vi "Autonomous.vi"   [LabVIEW 2019]
doc: "This VI starts when autonomous period begins, and will automatically be terminated when it ends. You can carry out timed or sensor driven operations directly to I/O or to subsystems without needing to return to the caller."
uses:
  <vilib>/Rock Robotics/WPI/Utilities/WPI_GetSetVariantRefNum.vi
  <vilib>/Rock Robotics/Network Tables/NT Read String.vi
types:
  T1 = typedef "WPI_JoystickDevRef.ctl" = cluster{"Device":T2}
  T2 = typedef "WPI_JoystickDeviceEnum.ctl" = enum16{"USB 0", "USB 1", "USB 2", "USB 3", "USB 4", "USB 5"}
  T3 = typedef "Command Status Info.ctl" = cluster{"Name":string, "Status":T4, "notifier out":T5}
  T4 = typedef "Completion Status.ctl" = enum16{"Successful", "Aborted", "Incomplete"}
  T5 = typedef "Completion Notifier.ctl" = refnum<notifier>
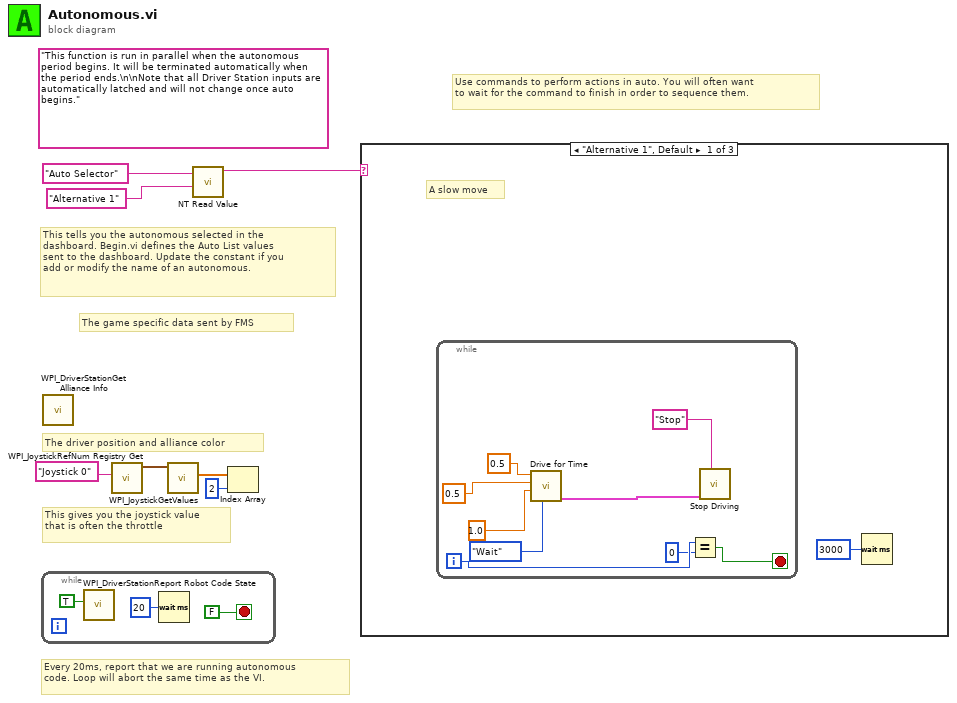
[diagram p0: block diagram]
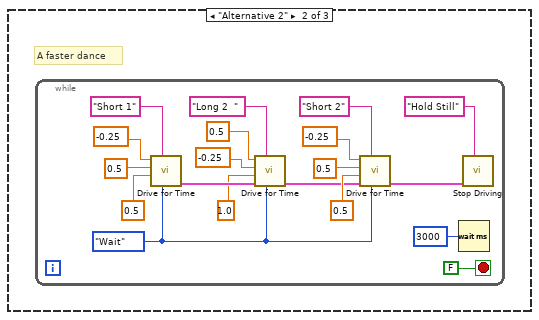
[diagram p2: hidden frame]
diagram:
  (unwired) "This function is run in parallel when the autonomous period begins. It will be terminated automatically when the period ends.\n\nNote that all Driver Station inputs are automatically latched and will not change once auto begins."
  # "The game specific data sent by FMS"
  # "This tells you the autonomous selected in the \ndashboard. Begin.vi defines the Auto List values\nsent to the dashboard. Update the constant if you\nadd or modify the name of an autonomous."
  # "Every 20ms, report that we are running autonomous\ncode. Loop will abort the same time as the VI."
  # "This gives you the joystick value\nthat is often the throttle"
  # "Use commands to perform actions in auto. You will often want\nto wait for the command to finish in order to sequence them."
  # "The driver position and alliance color"
  n1 = while {
    stop <- FALSE stop-if-true
    n2 = call <vilib>:"WPI_DriverStationReport Robot Code State.vi"("Autonomous"=TRUE) -> ()  [unwired: 10 in, 1 out]
    n3 = Wait (ms)(milliseconds to wait=u32 20) -> ()  [unwired: 1 out]
  }
  n4 = call <vilib>:"WPI_DriverStationGet Alliance Info.vi"() -> ()  [unwired: 12 out]
  n5 = call <vilib>:"WPI_JoystickRefNum Registry Get.vi"("refnum name"="Joystick 0") -> ("JoystickDevRef"=w6:T1)  [unwired: 1 in, 9 out]
  n6 = call <vilib>:"WPI_JoystickGetValues.vi"("JoystickDevRef"=w6) -> ("Axes"=w5:dbl[])  [unwired: 6 in, 4 out]
  n7 = call-poly <vilib>:"NT Read Value.vi"("Default Value"="Alternative 1", "Name"="Auto Selector") -> ("String"=w2:string)  [unwired: 8 in, 1 out]
  n8 = Index Array(array=w5, index=2) -> ()  [unwired: 1 out]
  n9 = case shown="\"Alternative 1\", Default" w2 {
    frame "Alternative 1", Default {
      # "A slow move"
      n10 = while {
        i -> [w14]
        stop <- w12 stop-if-true
        n11 = call "Drive for Time.vi"("Synchronization"=enum16{"Start", "Wait"}."Wait", "Seconds"=1.0, "Right Speed"=0.5, "Left Speed"=0.5) -> ("Command Info Out"=w20:T3)  [unwired: 7 in]
        n12 = Equal?(x=w14, y=0) -> (x = y?=w12:bool)
        n13 = call "Stop Driving.vi"("Description"="Stop", "Command Info In"=w20) -> ()  [unwired: 9 in, 1 out]
      }
      n14 = Wait (ms)(milliseconds to wait=u32 3000 ("millisecond timer value")) -> ()  [unwired: 1 out]
    }
    frame "Alternative 2" {
      # "A faster dance"
      n15 = while {
        stop <- FALSE stop-if-true
        w21 = enum16{"Start", "Wait"}."Wait" ("Synchronication")
        n16 = call "Drive for Time.vi"("Synchronization"=w21, "Description"="Short 1", "Seconds"=0.5 ("Delay (s)"), "Right Speed"=0.5 ("X axis value"), "Left Speed"=-0.25 ("X axis value")) -> ("Command Info Out"=w39:T3)  [unwired: 6 in]
        n17 = call "Drive for Time.vi"("Synchronization"=w21, "Description"="Long 2  ", "Command Info In"=w39, "Seconds"=1.0 ("Delay (s)"), "Right Speed"=-0.25 ("X axis value"), "Left Speed"=0.5 ("X axis value")) -> ("Command Info Out"=w23:T3)  [unwired: 5 in]
        n18 = call "Drive for Time.vi"("Synchronization"=w21, "Description"="Short 2", "Command Info In"=w23, "Seconds"=0.5 ("Delay (s)"), "Right Speed"=0.5 ("X axis value"), "Left Speed"=-0.25 ("X axis value")) -> ("Command Info Out"=w22:T3)  [unwired: 5 in]
        n19 = Wait (ms)(milliseconds to wait=u32 3000 ("millisecond timer value")) -> ()  [unwired: 1 out]
        n20 = call "Stop Driving.vi"("Description"="Hold Still", "Command Info In"=w22) -> ()  [unwired: 9 in, 1 out]
      }
    }
    frame "Your Turn" {
    }
  }
